vi "Get Channel.vi"   [LabVIEW 2011, in "labvvis.lvlib"]
doc: "Provides access to a channel in a RGBA image. Modifying the resultant \"image\" will actually modify the channel in the original image."
uses:
  <userlib>/labvvis/labvvis.lvlib
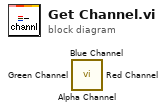
[diagram p0: block diagram]
diagram:
  n1 = call <userlib>:"Alpha Channel.vi"() -> ()  [unwired: 2 in, 2 out]
  n2 = call <userlib>:"Blue Channel.vi"() -> ()  [unwired: 2 in, 2 out]
  n3 = call <userlib>:"Green Channel.vi"() -> ()  [unwired: 2 in, 2 out]
  n4 = call <userlib>:"Red Channel.vi"() -> ()  [unwired: 2 in, 2 out]
